vi "WLAN - Test - UTIL - GenerateRxTVFilePath.vi"() -> (8 "RxMeasurementsCSV":path)   [LabVIEW 2011]
uses:
  <vilib>/Utility/file.llb/Write To Spreadsheet File (string).vi
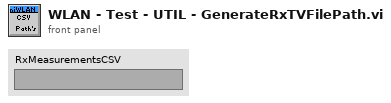
[diagram p1: front panel]
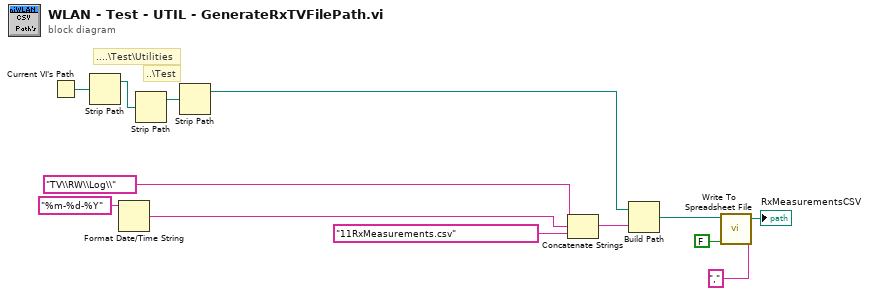
[diagram p0: block diagram]
diagram:
  # "....\\Test\\Utilities"
  # "..\\Test"
  n1 = Current VI's Path() -> (path=w13:path)
  n2 = Strip Path(path=w13) -> (stripped path=w12:path)  [unwired: 1 out]
  n3 = Format Date/Time String(time format string (%c)="%m-%d-%Y") -> (date/time string=w8:string)  [unwired: 2 in]
  n4 = Strip Path(path=w12) -> (stripped path=w11:path)  [unwired: 1 out]
  n5 = Strip Path(path=w11) -> (stripped path=w7:path)  [unwired: 1 out]
  n6 = Concatenate Strings("TV\\RW\\Log\\" ("name or relative path"), w8, "11RxMeasurements.csv" ("name or relative path")) -> (w5:string)
  n7 = Build Path(base path=w7, name or relative path=w5) -> (appended path=w2:path)
  n8 = call-poly <vilib>:"Write To Spreadsheet File.vi"("delimiter (\\t)"="," ("delimiter (\\t)"), "append to file? (new file:F)"=FALSE, "file path (dialog if empty)"=w2) -> ("new file path (Not A Path if cancelled)"=→"RxMeasurementsCSV":path)  [unwired: 5 in]
